vi "CoboltLaser_OutputPowerGet.vi"(0 "ComPort":refnum<visa-resource-name>, 7 "CheckResponse":bool=TRUE, 11 "ErrorIn":errorcluster) -> (4 "ComPortOut":refnum<visa-resource-name>, 6 "OutputPower":dbl format="%.4g", 15 "ErrorOut":errorcluster)   [LabVIEW 2019]
doc: "Use this template to build a VI to use as a subVI."
panel:
  out "ResponseOK":bool
  out "Response":string
  # "(W)"
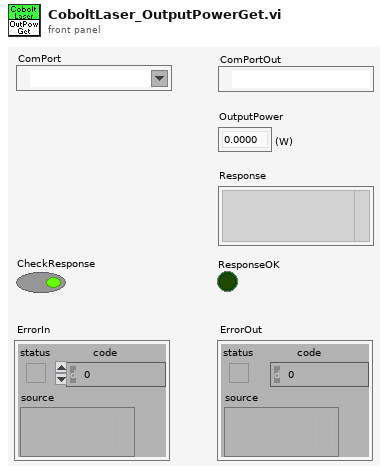
[diagram p1: front panel]
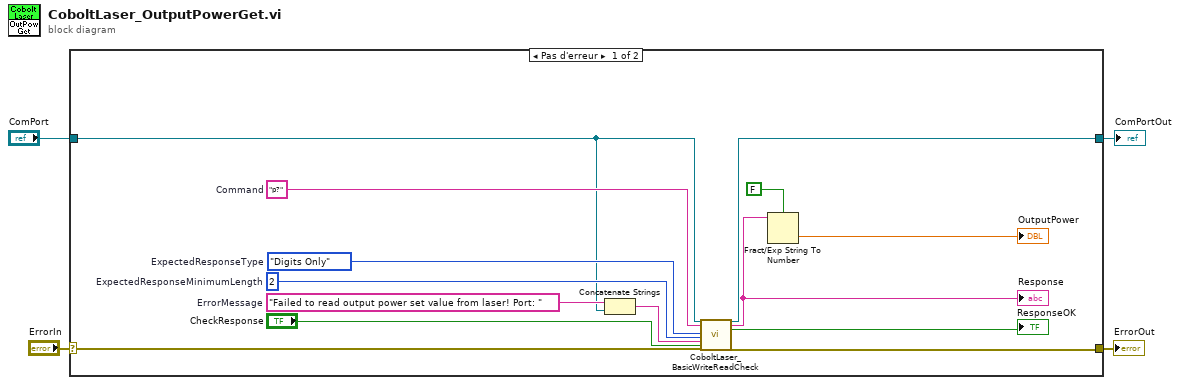
[diagram p0: block diagram]
diagram:
  n1 = case shown="Pas d'erreur" "ErrorIn" {
    selector: "ErrorIn" -> [w18 w20]
    tunnel: [w17 w20] -> w3
    tunnel: "ComPort" -> [w7 w19]
    tunnel: [w6 w19] -> w1
    frame No Error {
      w14 = 2  # ExpectedResponseMinimumLength
      w15 = enum16{"Any", "Digits Only", "Non-Digits Only"}."Digits Only"  # ExpectedResponseType
      w11 = "Failed to read output power set value from laser! Port: "  # ErrorMessage
      w16 = "p?"  # Command
      n2 = Concatenate Strings(w11, w7) -> (w10:string)
      n3 = call <userlib>:"CoboltLaser_BasicWriteReadCheck.vi"("ComPort"=w7, "Command"=w16, "ExpectedResponseType"=w15, "ExpectedResponseMinimumLength"=w14, "ErrorMessage"=w10, "GenerateError"="CheckResponse", "error in (no error)"=w18) -> ("ComPortOut"=w6:refnum<visa-resource-name>, "Response"=w9:string, "ResponseOK"=→"ResponseOK":bool, "error out"=w17:errorcluster)  [unwired: 17 in]
      "Response" <- w9
      n4 = Fract/Exp String To Number(use system decimal point (T)=FALSE, string=w9) -> (number=→"OutputPower":dbl)  [unwired: 2 in, 1 out]
    }
    frame Error {
    }
  }
  "ErrorOut" <- w3
  "ComPortOut" <- w1
